vi "A.vi"(1 "Promien krzywizny południka [v]":ext, 2 ">fi[rad]>":ext) -> (0 "A":ext)   [LabVIEW 2012, in "Biblioteka moduł map v3.lvlib" / "Konwersja wsp.lvlib" / "UTM.lvlib" / "Konwersja na UTM.lvlib"]
doc: "Współczynnik wzoru na konwersję na UTM."
uses:
  Konwersja na UTM.lvlib
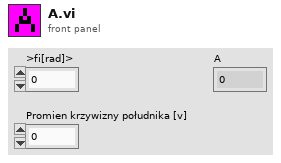
[diagram p1: front panel]
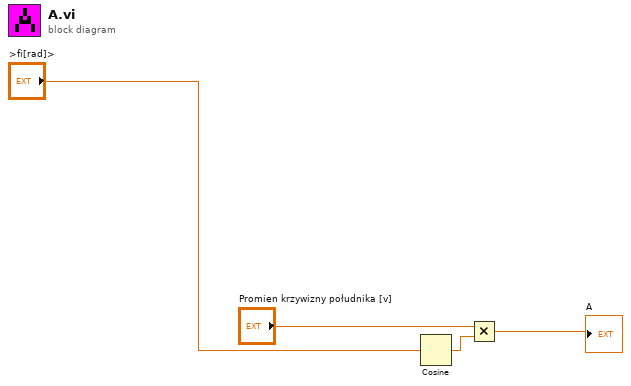
[diagram p0: block diagram]
diagram:
  n1 = Cosine(x=">fi[rad]>") -> (cos(x)=w3:ext)
  n2 = Multiply(x="Promien krzywizny południka [v]", y=w3) -> (x*y=→"A":ext)
